vi "IMAQController.Write To Spreadsheet File (DBL).vi"(0 "file path (dialog if empty)":path, 1 "Column Header":dbl[](array[numeric]) format="%0.2f", 2 "2D data":dbl[][](array[numeric]) format="%0.2f", 3 "1D data":dbl[](array[numeric]) format="%0.2f", 4 "General Header":string="%.3f", 5 "Row Header":dbl[](array[numeric]) format="%0.2f", 6 "format (%.3f)":string="%.3f", 7 "append to file? (new file:F)":bool, 9 "transpose? (no:F)":bool, 11 "delimiter (\\t)":string="\t") -> (14 "new file path (Not A Path if cancelled)":path)   [LabVIEW 2014, in "IMAQController.lvlib"]
doc: "Converts a 2D or 1D array of strings, signed integers, or double-precision numbers to a text string and writes the string to a new byte stream file or appends the string to an existing file. Wire data to the <B>2D data</B> input or <B>1D data</B> input to determine the polymorphic instance to use or manually select the instance.\n\nUse this VI to transpose or separate data.\n\n<B>Note</B> To format with Microsoft Excel, use ActiveX with LabVIEW or the Report Generation Toolkit for Microsoft Office."
uses:
  IMAQController.lvlib
  <vilib>/Utility/error.llb/DialogType.ctl
panel:
  in  "prompt":string="Choose file to write."
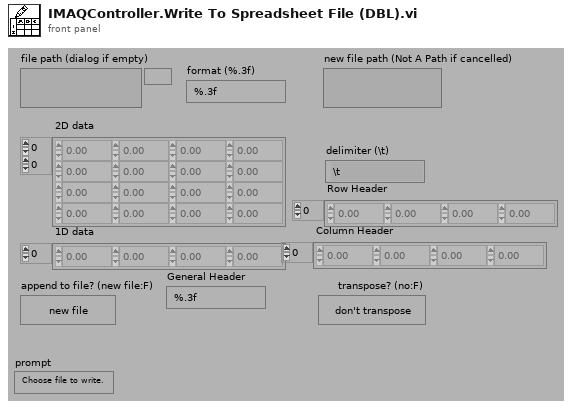
[diagram p1: front panel]
types:
  T1 = typedef "DialogType.ctl" = u16
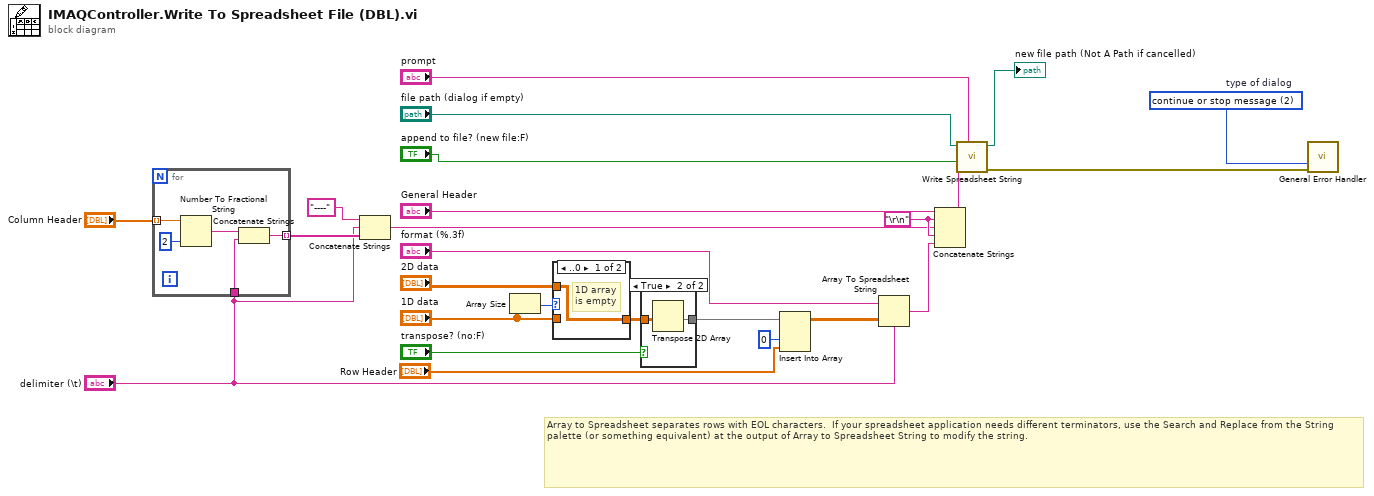
[diagram p0: block diagram]
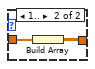
[diagram p3: hidden frame]
diagram:
  w11 = "\r\n"
  w14 = T1 2 items=["no dialog", "OK message", "continue or stop message", "OK message + warnings", "continue/stop + warnings"]  # type of dialog
  # "Array to Spreadsheet separates rows with EOL characters.  If your spreadsheet application needs different terminators, use the Search and Replace from the String palette (or something equivalent) at the output of Array to Spreadsheet String to modify the string."
  n1 = for {
    tunnel: "Column Header" -> [w30] mode=indexing
    tunnel: "delimiter (\\t)" -> [w27]
    tunnel: [w26] -> w4 mode=indexing
    n2 = Number To Fractional String(number=w30, precision (6)=i16 2) -> (F-format string=w28:string)  [unwired: 2 in]
    n3 = Concatenate Strings(w28, w27) -> (w26:string)
  }
  n4 = Concatenate Strings("----" ("string"), "delimiter (\\t)", w4) -> (w3:string)
  n5 = Array Size(array="1D data") -> (size(s)=w24:i32)
  n6 = case shown="..0" w24 {
    tunnel: "1D data" -> [_ w33]
    tunnel: [w31 w32] -> w20
    tunnel: "2D data" -> [w31 _]
    frame ..0 {
      # "1D array is empty"
    }
    frame 1.. {
      n7 = Build Array(w33) -> (w32:dbl[][])
    }
  }
  n8 = case shown="True" "transpose? (no:F)" {
    tunnel: [w34 w36] -> w6
    tunnel: w20 -> [w34 w35]
    frame False {
    }
    frame True {
      n9 = Transpose 2D Array(2D array=w35) -> (transposed array=w36:dbl[][])
    }
  }
  n10 = Insert Into Array(array=w6, index (col)=0 ("disabled index (col)"), new element="Row Header") -> (w7:dbl[][])  [unwired: 1 in]
  n11 = Array To Spreadsheet String(delimiter (Tab)="delimiter (\\t)", array=w7, 3:"format (%.3f)") -> (spreadsheet string=w10:string)
  n12 = Concatenate Strings("General Header", w11, w3, w11, w10) -> (w13:string)
  n13 = call <vilib>:"Write Spreadsheet String.vi"("prompt"="prompt", "append to file? (new file:F)"="append to file? (new file:F)", "spreadsheet string"=w13, "file path (dialog if empty)"="file path (dialog if empty)") -> ("error out"=w15:errorcluster, "path"=→"new file path (Not A Path if cancelled)":path)  [unwired: 6 in]
  n14 = call <vilib>:"General Error Handler.vi"("type of dialog (OK msg:1)"=w14, "error in (no error)"=w15) -> ()  [unwired: 9 in, 5 out]
